vi "Combination_Digitizer_Driver.vi"(0 "Mode":T1(ring), 1 "Horizontal Settings":T2={"number of records"=1, "reference position"=50.0, "min record length"=50000, "min sample rate"=200000.0, "enforce realtime"=FALSE, "maximum input frequency"=0.0} {"maximum input frequency" format="%.2f"; "min sample rate" step=1000000.0; "reference position" format="%.1f"; "number of records" step=1}, 2 "Vertical Settings":T4={"vertical coupling"=enum."DC", "probe attenuation"=20.0, "vertical range"=120.0, "vertical offset"=0.0} {"vertical offset" format="%.4f"; "vertical range" format="%.2f"; "probe attenuation" format="%.1f"}, 3 "Trigger settings":T3={"trigger level"=30.0, "trigger type"=enum."Edge", "Trigger Source"=enum."Channel 0", "Trigger Slope"=enum."Positive"} {"trigger level" format="%.2f"}, 5 "Channel Name":string="0", 11 "error in":errorcluster) -> (6 "Waveform Array":waveform(dbl)[](array[waveform]), 8 "Ch1_Plot":dbl[](array[numeric]), 15 "error out":errorcluster)   [LabVIEW 2010]
uses:
  <instrlib>/niScope/Acquire/niScope Multi Read Cluster.vi
panel:
  out "Waveform":T5(graph)
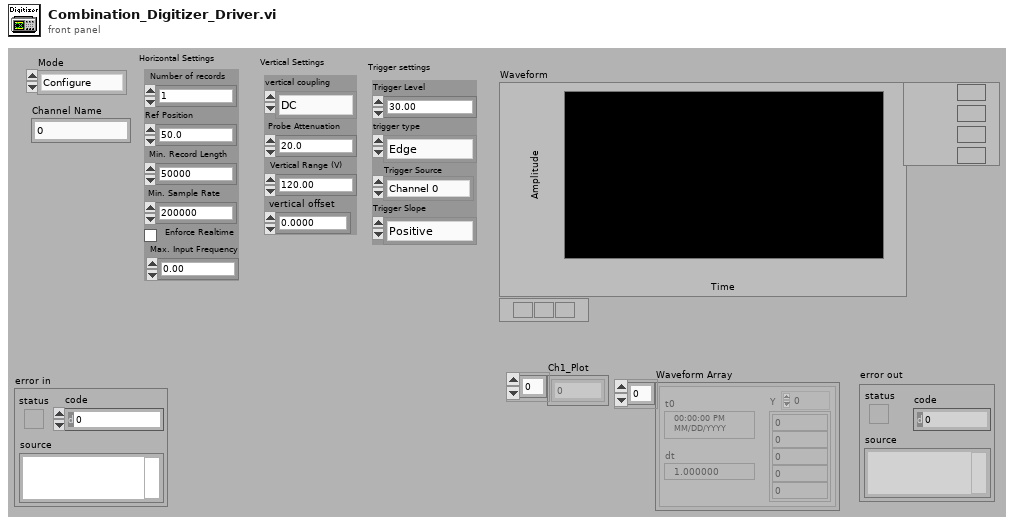
[diagram p1: front panel]
types:
  T1 = enum16{"Configure", "Read", "TriggerRead", "Close", "Init"}
  T2 = cluster{"number of records":i32, "reference position":dbl, "min record length":i32, "min sample rate":dbl, "enforce realtime":bool, "maximum input frequency":dbl}
  T3 = cluster{"trigger level":dbl, "trigger type":enum16{"Edge", "Digital", "Immediate"}, "Trigger Source":enum8{"Immediate", "Channel 0", "Channel 1", "Channel 2", "Channel 3", "Channel 4", "Channel 5", "Channel 6", "Channel 7", "External TRIG", "Software Trigger", "RTSI 0", "RTSI 1", "RTSI 2", "RTSI 3", "RTSI 4", "RTSI 5", "RTSI 6", "PFI 0", "PFI 1", "PFI 2", "PXI Star Trigger"}, "Trigger Slope":enum16{"Positive", "Negative"}}
  T4 = cluster{"vertical coupling":enum16{"AC", "DC", "Ground"}, "probe attenuation":dbl, "vertical range":dbl, "vertical offset":dbl}
  T5 = cluster{"relativeInitialX":dbl, "xIncrement":dbl, "wfm":dbl[]}[]
  T6 = cluster{"Dig1 Channels":string, "Channel1 Scale":dbl, "Dig1 Used":bool, "Dig1 Ref":refnum<k15>, "min record length":i32, "Dig2 Channels":string, "Dig2 Used":bool, "Dig2 Ref":refnum<k15>, "trigger type":enum16{"Edge", "Digital", "Immediate"}}
  T7 = cluster{"relativeInitialX":dbl, "xIncrement":dbl, "wfm":dbl[]}
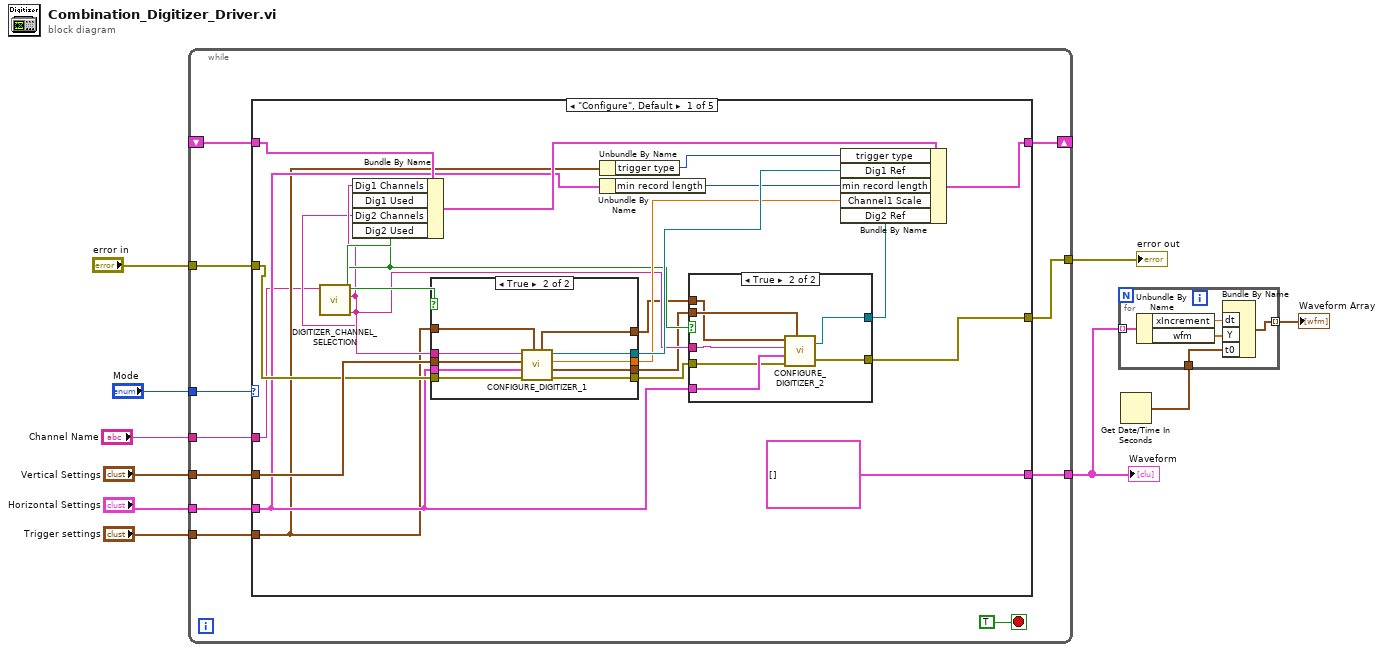
[diagram p0: block diagram]
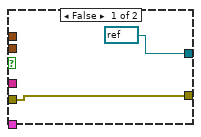
[diagram p2: hidden frame]
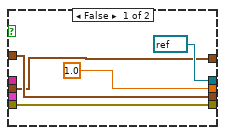
[diagram p3: hidden frame]
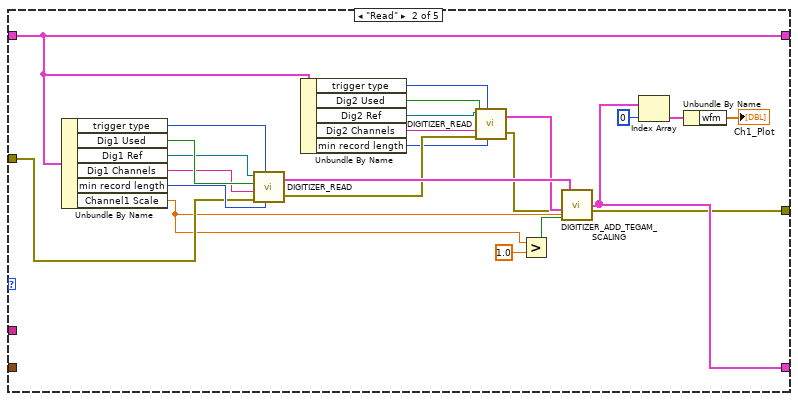
[diagram p4: hidden frame]
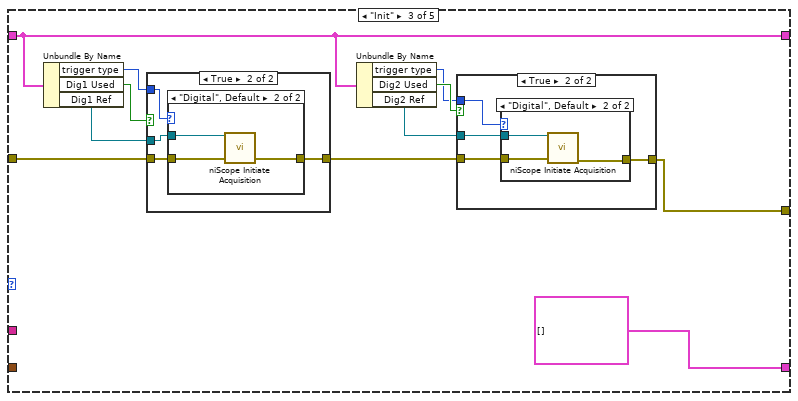
[diagram p5: hidden frame]
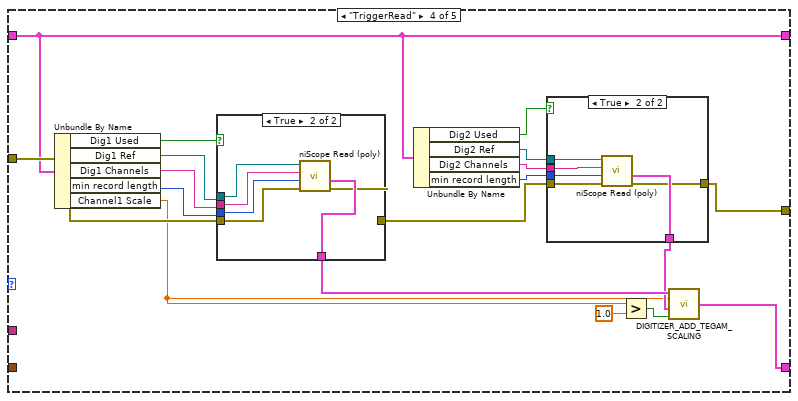
[diagram p10: hidden frame]
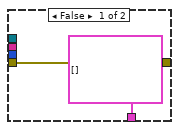
[diagram p11: hidden frame]
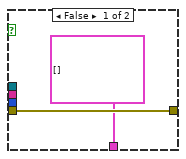
[diagram p12: hidden frame]
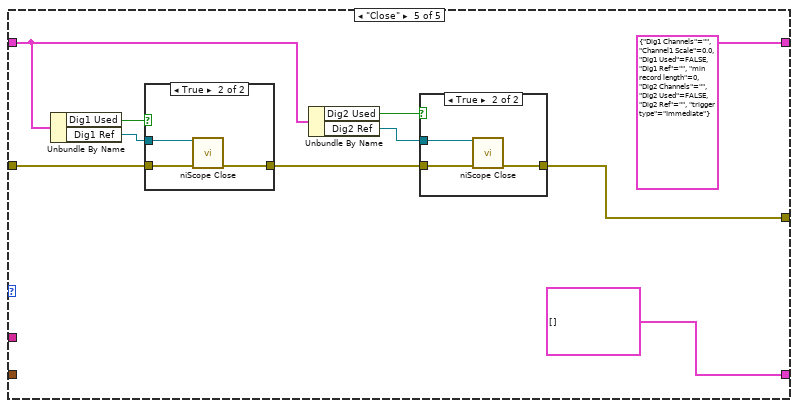
[diagram p13: hidden frame]
diagram:
  n1 = while {
    tunnel: "Mode" -> [w20]
    shift-right: [w14] -> _
    shift-left: _ -> [w19]
    tunnel: "error in" -> [w13]
    tunnel: "Channel Name" -> [w18]
    tunnel: "Vertical Settings" -> [w17]
    tunnel: "Horizontal Settings" -> [w16]
    tunnel: "Trigger settings" -> [w15]
    tunnel: [w12] -> w5
    tunnel: [w11] -> w3
    stop <- TRUE stop-if-true
    n2 = case shown="\"Configure\", Default" w20 {
      tunnel: w19 -> [w39 w81 w94 w125 w156]
      tunnel: w18 -> [w22 _ _ _ _]
      tunnel: w17 -> [w42 _ _ _ _]
      tunnel: w16 -> [w29 _ _ _ _]
      tunnel: w15 -> [w26 _ _ _ _]
      tunnel: [w41 w81 w94 w125 T6 {"Dig1 Channels"="", "Channel1 Scale"=0.0, "Dig1 Used"=FALSE, "Dig1 Ref"="", "min record length"=0, "Dig2 Channels"="", "Dig2 Used"=FALSE, "Dig2 Ref"="", "trigger type"=enum."Immediate"}] -> w14
      tunnel: w13 -> [w40 w83 w97 w130 w159]
      tunnel: [w34 w74 w100 w135 w162] -> w12
      tunnel: [T5 [] w79 T5 [] w120 T5 []] -> w11
      frame "Configure", Default {
        n3 = call "DIGITIZER_CHANNEL_SELECTION.vi"("Channel Name"=w22) -> ("DIGITIZER 2 CHANNELS"=w30:string, "DIGITIZER 2 USED?"=w32:bool, "DIGITIZER 1 CHANNELS"=w31:string, "DIGITIZER 1 USED?"=w33:bool)  [unwired: 4 in, 1 out]
        n4 = Bundle By Name(cluster=w39, "Dig1 Channels"=w31, "Dig1 Used"=w33, "Dig2 Channels"=w30, "Dig2 Used"=w32) -> (w38:T6)
        n5 = case shown="True" w33 {
          tunnel: [w57 w67] -> w43
          tunnel: w40 -> [w57 w66]
          tunnel: w31 -> [_ w58]
          tunnel: w42 -> [w53 w60]
          tunnel: w29 -> [_ w65]
          tunnel: w26 -> [w54 w62]
          tunnel: [refnum<k15> refnum ("instrument handle out") w64] -> w37
          tunnel: [1.0 ("Gain Multiplier") w63] -> w35
          tunnel: [w54 w61] -> w24
          tunnel: [w53 w59] -> w23
          frame False {
          }
          frame True {
            n6 = call "CONFIGURE_DIGITIZER_1.vi"("TRIGGER SETTINGS IN"=w62, "error in"=w66, "Horizontal Settings IN"=w65, "Vertical Settings IN"=w60, "DIGITIZER 1 CHANNELS"=w58) -> ("error out"=w67:errorcluster, "TRIGGER SETTINGS OUT"=w61:T3, "Gain Multiplier"=w63:dbl, "instrument handle out"=w64:refnum<k15>, "VERTICAL SETTINGS OUT"=w59:T4)
          }
        }
        n7 = Unbundle By Name(w26) -> ("trigger type"=w25:enum16{"Edge", "Digital", "Immediate"})
        n8 = Unbundle By Name(w29) -> ("min record length"=w28:i32)
        n9 = case shown="True" w32 {
          tunnel: [w45 w48] -> w34
          tunnel: w43 -> [w45 w50]
          tunnel: w30 -> [_ w46]
          tunnel: w29 -> [_ w52]
          tunnel: w24 -> [_ w51]
          tunnel: [refnum<k15> refnum ("instrument handle out") w49] -> w36
          tunnel: w23 -> [_ w47]
          frame False {
          }
          frame True {
            n10 = call "CONFIGURE_DIGITIZER_2.vi"("VERTICAL SETTINGS IN"=w47, "DIGITIZER 2 CHANNELS"=w46, "Horizontal Settings IN"=w52, "error in"=w50, "TRIGGER SETTINGS IN"=w51) -> ("instrument handle out"=w49:refnum<k15>, "error out"=w48:errorcluster)
          }
        }
        n11 = Bundle By Name(cluster=w38, "trigger type"=w25, "Dig1 Ref"=w37, "min record length"=w28, "Channel1 Scale"=w35, "Dig2 Ref"=w36) -> (w41:T6)
      }
      frame "Read" {
        n12 = Unbundle By Name(w81) -> ("trigger type"=w76:enum16{"Edge", "Digital", "Immediate"}, "Dig1 Used"=w87:bool, "Dig1 Ref"=w86:refnum<k15>, "Dig1 Channels"=w85:string, "min record length"=w84:i32, "Channel1 Scale"=w82:dbl)
        n13 = call "DIGITIZER_READ.vi"("min record length"=w84, "trigger type"=w76, "error in"=w83, "DIG CHANNELS"=w85, "DIG USED?"=w87, "DIG REF"=w86) -> ("error out"=w73:errorcluster, "waveform"=w88:T5)
        n14 = Unbundle By Name(w81) -> ("trigger type"=w72:enum16{"Edge", "Digital", "Immediate"}, "Dig2 Used"=w71:bool, "Dig2 Ref"=w70:refnum<k15>, "Dig2 Channels"=w69:string, "min record length"=w68:i32)
        n15 = call "DIGITIZER_READ.vi"("min record length"=w68, "trigger type"=w72, "error in"=w73, "DIG CHANNELS"=w69, "DIG USED?"=w71, "DIG REF"=w70) -> ("error out"=w74:errorcluster, "waveform"=w75:T5)
        n16 = Greater?(x=w82, y=1.0) -> (0:w90:bool)
        n17 = call "DIGITIZER_ADD_TEGAM_SCALING.vi"("TEGAM SCALING PRESENT?"=w90, "DIGITIZER 2 WAVEFORM"=w75, "Channel1 Scale"=w82, "DIGITIZER 1 WAVEFORM"=w88) -> ("WAVEFORMS OUT"=w79:T5)
        n18 = Index Array(array=w79, index=0) -> (element=w78:T7)
        n19 = Unbundle By Name(w78) -> ("wfm"=→"Ch1_Plot":dbl[])
      }
      frame "Init" {
        n20 = Unbundle By Name(w94) -> ("trigger type"=w93:enum16{"Edge", "Digital", "Immediate"}, "Dig1 Used"=w99:bool, "Dig1 Ref"=w98:refnum<k15>)
        n21 = case shown="True" w99 {
          tunnel: w97 -> [w111 w114]
          tunnel: w98 -> [_ w115]
          tunnel: [w111 w113] -> w101
          tunnel: w93 -> [_ w112]
          frame False {
          }
          frame True {
            n22 = case shown="\"Digital\", Default" w112 {
              tunnel: w115 -> [_ w118]
              tunnel: w114 -> [w116 w117]
              tunnel: [w116 w119] -> w113
              frame "Immediate" {
              }
              frame "Digital", Default {
                n23 = call <instrlib>:"niScope Initiate Acquisition.vi"("instrument handle"=w118, "error in"=w117) -> ("error out"=w119:errorcluster)  [unwired: 12 in, 1 out]
              }
            }
          }
        }
        n24 = Unbundle By Name(w94) -> ("trigger type"=w92:enum16{"Edge", "Digital", "Immediate"}, "Dig2 Used"=w96:bool, "Dig2 Ref"=w95:refnum<k15>)
        n25 = case shown="True" w96 {
          tunnel: w101 -> [w102 w104]
          tunnel: w95 -> [_ w105]
          tunnel: [w102 w106] -> w100
          tunnel: w92 -> [_ w103]
          frame False {
          }
          frame True {
            n26 = case shown="\"Digital\", Default" w103 {
              tunnel: w105 -> [_ w109]
              tunnel: w104 -> [w107 w108]
              tunnel: [w107 w110] -> w106
              frame "Immediate" {
              }
              frame "Digital", Default {
                n27 = call <instrlib>:"niScope Initiate Acquisition.vi"("instrument handle"=w109, "error in"=w108) -> ("error out"=w110:errorcluster)  [unwired: 12 in, 1 out]
              }
            }
          }
        }
      }
      frame "TriggerRead" {
        n28 = Unbundle By Name(w125) -> ("Dig1 Used"=w134:bool, "Dig1 Ref"=w133:refnum<k15>, "Dig1 Channels"=w132:string, "min record length"=w131:i32, "Channel1 Scale"=w121:dbl)
        n29 = case shown="True" w134 {
          tunnel: w132 -> [_ w152]
          tunnel: w130 -> [w147 w153]
          tunnel: w133 -> [_ w151]
          tunnel: [w147 w148] -> w136
          tunnel: [T5 [] ("waveform") w150] -> w124
          tunnel: w131 -> [_ w149]
          frame False {
          }
          frame True {
            n30 = call-poly <instrlib>:"niScope Read (poly).vi"("error in"=w153, "numSamples"=w149, "channels"=w152, "instrument handle"=w151) -> ("error out"=w148:errorcluster, "waveform"=w150:T5)  [unwired: 4 in, 2 out]
          }
        }
        n31 = Unbundle By Name(w125) -> ("Dig2 Used"=w129:bool, "Dig2 Ref"=w128:refnum<k15>, "Dig2 Channels"=w127:string, "min record length"=w126:i32)
        n32 = case shown="True" w129 {
          tunnel: w127 -> [_ w144]
          tunnel: w136 -> [w139 w145]
          tunnel: w128 -> [_ w143]
          tunnel: w126 -> [_ w142]
          tunnel: [w139 w140] -> w135
          tunnel: [T5 [] ("waveform") w141] -> w122
          frame False {
          }
          frame True {
            n33 = call-poly <instrlib>:"niScope Read (poly).vi"("error in"=w145, "numSamples"=w142, "channels"=w144, "instrument handle"=w143) -> ("error out"=w140:errorcluster, "waveform"=w141:T5)  [unwired: 4 in, 2 out]
          }
        }
        n34 = Greater?(x=w121, y=1.0) -> (0:w123:bool)
        n35 = call "DIGITIZER_ADD_TEGAM_SCALING.vi"("TEGAM SCALING PRESENT?"=w123, "DIGITIZER 2 WAVEFORM"=w122, "Channel1 Scale"=w121, "DIGITIZER 1 WAVEFORM"=w124) -> ("WAVEFORMS OUT"=w120:T5)
      }
      frame "Close" {
        n36 = Unbundle By Name(w156) -> ("Dig1 Used"=w161:bool, "Dig1 Ref"=w160:refnum<k15>)
        n37 = case shown="True" w161 {
          tunnel: w159 -> [w168 w169]
          tunnel: w160 -> [_ w170]
          tunnel: [w168 w171] -> w163
          frame False {
          }
          frame True {
            n38 = call <instrlib>:"niScope Close.vi"("instrument handle"=w170, "error in"=w169) -> ("error out"=w171:errorcluster)  [unwired: 13 in]
          }
        }
        n39 = Unbundle By Name(w156) -> ("Dig2 Used"=w158:bool, "Dig2 Ref"=w157:refnum<k15>)
        n40 = case shown="True" w158 {
          tunnel: w163 -> [w164 w166]
          tunnel: w157 -> [_ w165]
          tunnel: [w164 w167] -> w162
          frame False {
          }
          frame True {
            n41 = call <instrlib>:"niScope Close.vi"("instrument handle"=w165, "error in"=w166) -> ("error out"=w167:errorcluster)  [unwired: 13 in]
          }
        }
      }
    }
  }
  "error out" <- w5
  "Waveform" <- w3
  n42 = Get Date/Time In Seconds() -> (seconds since 1Jan1904=w1:timestamp)
  n43 = for {
    tunnel: w3 -> [w176] mode=indexing
    tunnel: [w173] -> w2 mode=indexing
    tunnel: w1 -> [w172]
    n44 = Unbundle By Name(w176) -> ("xIncrement"=w175:dbl, "wfm"=w174:dbl[])
    n45 = Bundle By Name("dt"=w175, "Y"=w174, "t0"=w172) -> (w173:waveform(dbl))  [unwired: 1 in]
  }
  "Waveform Array" <- w2
